vi "input.vi"(1 "INPUT":T1) -> (0 "OUTPUT":T2)   [LabVIEW 2013]
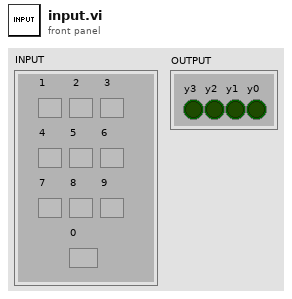
[diagram p1: front panel]
types:
  T1 = cluster{"1":bool, " 2":bool, " 3":bool, "4":bool, "5":bool, "6":bool, "7":bool, "8":bool, "9":bool, "0":bool}
  T2 = cluster{"y0":bool, "y1":bool, "y2":bool, "y3":bool}
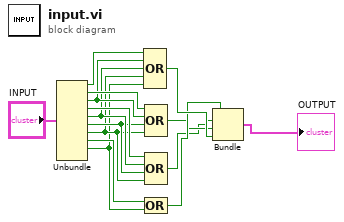
[diagram p0: block diagram]
diagram:
  n1 = Unbundle("INPUT") -> ("1"=w14:bool, "2"=w13:bool, "3"=w12:bool, "4"=w11:bool, "5"=w10:bool, "6"=w9:bool, "7"=w8:bool, "8"=w7:bool, "9"=w6:bool)  [unwired: 1 out]
  n2 = Compound Arithmetic op=OR(w14, w12, w10, w8, w6) -> (w4:bool)
  n3 = Compound Arithmetic op=OR(w13, w12, w9, w8) -> (w2:bool)
  n4 = Compound Arithmetic op=OR(w11, w10, w9, w8) -> (w1:bool)
  n5 = Compound Arithmetic op=OR(w7, w6) -> (w3:bool)
  n6 = Bundle(w3, w1, w2, w4) -> (→"OUTPUT":cluster{bool, bool, bool, bool})  [unwired: 1 in]
